vi "Excel_Set_Chart_Gridelines.vi"(0 "Axes in":refnum<k7>, 1 "gridlines":T1, 5 "Type":i32(ring)=1 items=["xlCategory"=1, "xlSeriesAxis"=3, "xlValue"=2], 11 "error in (no error)":errorcluster) -> (4 "Axes out":refnum<k7>, 15 "error out":errorcluster)   [LabVIEW 2020, in "NI_ReportGenerationToolkit.lvlib"]
uses:
  <vilib>/addons/_office/NI_ReportGenerationToolkit.lvlib
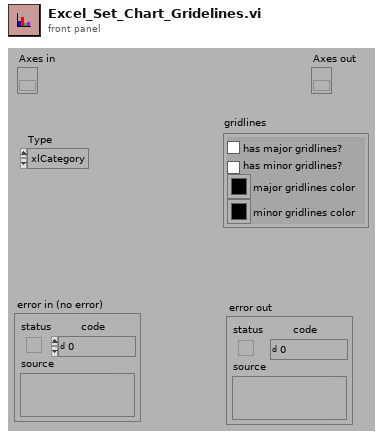
[diagram p1: front panel]
types:
  T1 = cluster{"has major gridlines?":bool, "has minor gridlines?":bool, "major gridlines color":u32, "minor gridlines color":u32}
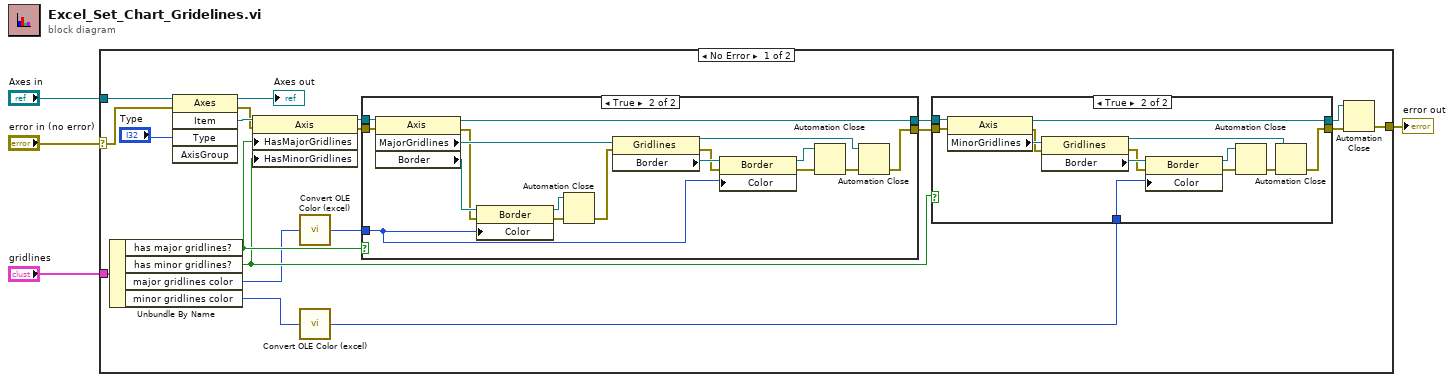
[diagram p0: block diagram]
diagram:
  n1 = case shown="No Error" "error in (no error)" {
    selector: "error in (no error)" -> [w6 w59]
    tunnel: "Axes in" -> [w24 _]
    tunnel: [w12 w59] -> w3
    tunnel: "gridlines" -> [w11 _]
    frame No Error {
      n2 = Unbundle By Name(w11) -> ("has major gridlines?"=w10:bool, "has minor gridlines?"=w9:bool, "major gridlines color"=w8:u32, "minor gridlines color"=w7:u32)
      n3 = invoke class="Axes" method="Item"(reference=w24, error in=w6, "Type"="Type") -> (reference out=→"Axes out":refnum<k7>, error out=w20:errorcluster, "Item"=w22:refnum<k7>)  [unwired: 2 in, 2 out]
      n4 = property class="Axis"(reference=w22, error in=w20, "HasMajorGridlines"=w10, "HasMinorGridlines"=w9) -> (reference out=w21:refnum<k7>, error out=w19:errorcluster)
      n5 = call <vilib>:"Convert OLE Color (excel).vi"("color in"=w8) -> ("color out"=w5:u32)
      n6 = call <vilib>:"Convert OLE Color (excel).vi"("color in"=w7) -> ("color out"=w16:u32)
      n7 = case shown="True" w10 {
        tunnel: w21 -> [w41 w58]
        tunnel: [w41 w51] -> w18
        tunnel: [w40 w50] -> w17
        tunnel: w19 -> [w40 w49]
        tunnel: w5 -> [_ w42]
        frame False {
        }
        frame True {
          n8 = property class="Axis"(reference=w58, error in=w49) -> (reference out=w51:refnum<k7>, error out=w45:errorcluster, "MajorGridlines"=w56:refnum<k7>, "Border"=w46:refnum<k7>)
          n9 = property class="Border"(reference=w46, error in=w45, "Color"=w42) -> (reference out=w44:refnum<k7>, error out=w47:errorcluster)
          n10 = Automation Close(3:w47, 5:w44) -> (0:w43:errorcluster)
          n11 = property class="Gridlines"(reference=w56, error in=w43) -> (reference out=w52:refnum<k7>, error out=w48:errorcluster, "Border"=w57:refnum<k7>)
          n12 = property class="Border"(reference=w57, error in=w48, "Color"=w42) -> (reference out=w54:refnum<k7>, error out=w55:errorcluster)
          n13 = Automation Close(3:w55, 5:w54) -> (0:w53:errorcluster)
          n14 = Automation Close(3:w53, 5:w52) -> (0:w50:errorcluster)
        }
      }
      n15 = case shown="True" w9 {
        tunnel: w18 -> [w26 w39]
        tunnel: [w26 w32] -> w13
        tunnel: [w25 w31] -> w14
        tunnel: w17 -> [w25 w30]
        tunnel: w16 -> [_ w27]
        frame False {
        }
        frame True {
          n16 = property class="Axis"(reference=w39, error in=w30) -> (reference out=w32:refnum<k7>, error out=w29:errorcluster, "MinorGridlines"=w37:refnum<k7>)
          n17 = property class="Gridlines"(reference=w37, error in=w29) -> (reference out=w33:refnum<k7>, error out=w28:errorcluster, "Border"=w38:refnum<k7>)
          n18 = property class="Border"(reference=w38, error in=w28, "Color"=w27) -> (reference out=w35:refnum<k7>, error out=w36:errorcluster)
          n19 = Automation Close(3:w36, 5:w35) -> (0:w34:errorcluster)
          n20 = Automation Close(3:w34, 5:w33) -> (0:w31:errorcluster)
        }
      }
      n21 = Automation Close(3:w14, 5:w13) -> (0:w12:errorcluster)
    }
    frame Error {
    }
  }
  "error out" <- w3
